vi "General-GetGaussianArray.vi"(0 "tiempo (ms)":dbl, 1 "Amplitud":dbl, 2 "t0 (ms)":dbl, 3 "Sigma (ms)":dbl, 4 "#samples":u32) -> (5 "Y out":dbl[](array[numeric]), 6 "t out":sgl[](array[numeric]))   [LabVIEW 2010]
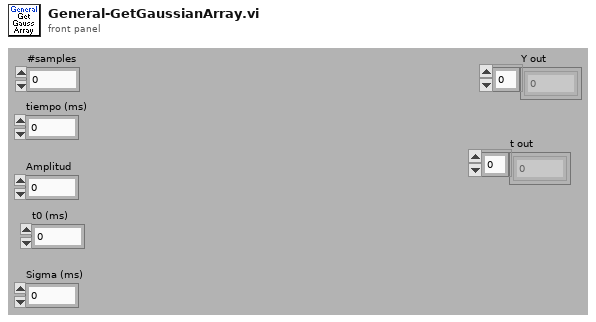
[diagram p1: front panel]
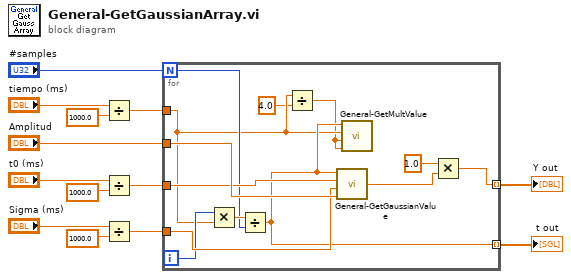
[diagram p0: block diagram]
diagram:
  n1 = Divide(x="tiempo (ms)", y=sgl 1000.0) -> (x/y=w1:dbl)
  n2 = Divide(x="t0 (ms)", y=sgl 1000.0) -> (x/y=w9:dbl)
  n3 = Divide(x="Sigma (ms)", y=sgl 1000.0) -> (x/y=w10:dbl)
  n4 = for {
    N: "#samples" -> [w22]
    tunnel: [w19] -> w11 mode=indexing
    tunnel: "Amplitud" -> [w25]
    tunnel: w10 -> [w24]
    tunnel: w9 -> [w23]
    tunnel: w1 -> [w17]
    tunnel: [w18] -> w13 mode=indexing
    i -> [w21]
    n5 = Multiply(x=w21, y=w17) -> (x*y=w26:dbl)
    n6 = Divide(x=w26, y=w22) -> (x/y=w18:dbl)
    n7 = Divide(x=w17, y=4.0) -> (x/y=w15:dbl)
    n8 = call "General-GetGaussianValue.vi"("Amplitud"=w25, "sigma"=w24, "miu"=w23, "x"=w18) -> ("out"=w20:dbl)
    n9 = call "General-GetMultValue.vi"("Ultimo Intervalo"=w15, "Primer Intervalo"=w15, "Tiempo Final"=w17, "t"=w18) -> ()  [unwired: 1 out]
    n10 = Multiply(x=1.0, y=w20) -> (x*y=w19:dbl)
  }
  "t out" <- w13
  "Y out" <- w11
